vi "Climber_Execute.vi"() -> ()   [LabVIEW 2020]
uses:
  Climber_Outer_Arm_Enum.ctl
  Climber_Inner_Arm_Enum.ctl
  <vilib>/Rock Robotics/WPI/Solenoid/WPI_SolenoidValue.ctl
  <vilib>/Rock Robotics/WPI/DriverStation/WPI_DriverStationRobotMode2.ctl
  Climber_Cluster.ctl
  Climber_Control_States.ctl
  Globals/Climber_Globals.vi
  Globals/Sensor_Values.vi
  Globals/Calibration_And_Constant_Globals.vi
  Robot Global Data.vi
panel:
  out "inner arm pivot command":T1
  out "outer arm pivot command":T2
  out "elevator command":dbl=-1.0 format="%_4g"
  out "elevator Current Error":dbl=-236249.0 format="%_4g"
  in  "Outer_Arm_Elevator_Goal":dbl(slide) scale=0.0..354000.0
  in  "acceptable outer arm elevator error":dbl=3000.0
  in  "Zero_PID":T3={"Kp"=0.0, "Ki"=0.0, "Kd"=0.0, "N-Diff"=10, "N-Int"=20, "Int Error Window"=0.5, "Max Ouput"=1.0, "Min Output"=-1.0} {"Int Error Window" min=0.0; "N-Int" min=2; "N-Diff" min=2; "Kd" min=0.0; "Ki" min=0.0; "Kp" min=0.0}
  in  "Outer_Elevator_No_Load":T3={"Kp"=3e-05, "Ki"=0.0, "Kd"=0.0, "N-Diff"=10, "N-Int"=20, "Int Error Window"=0.5, "Max Ouput"=1.0, "Min Output"=-1.0} {"Int Error Window" min=0.0; "N-Int" min=2; "N-Diff" min=2; "Kd" min=0.0; "Ki" min=0.0; "Kp" min=0.0}
  in  "Disable_Outer_Arm_Elevator_Limit_Safeties":bool
  in  "Outer_Arm_Elevator_Lower_Limit":dbl
  in  "Outer_Arm_Elevator_Upper_Limit":dbl=354000.0
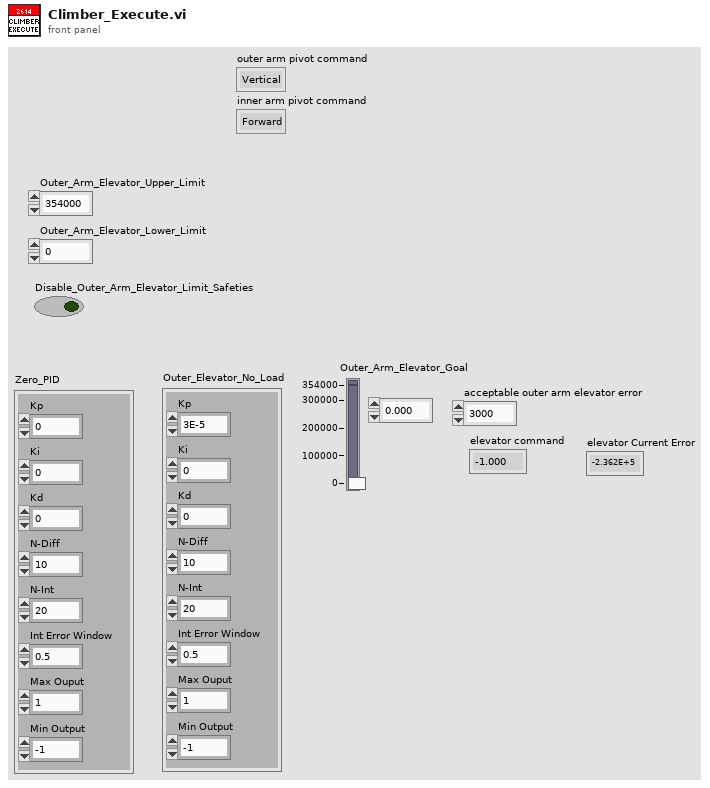
[diagram p1: front panel]
types:
  T1 = typedef "Climber_Inner_Arm_Enum.ctl" = enum16{"Forward", "Back"}
  T2 = typedef "Climber_Outer_Arm_Enum.ctl" = enum16{"Vertical", "Back"}
  T3 = cluster{"Kp":dbl, "Ki":dbl, "Kd":dbl, "N-Diff":i32, "N-Int":i32, "Int Error Window":dbl, "Max Ouput":dbl, "Min Output":dbl}
  T4 = typedef "WPI_DriverStationRobotMode2.ctl" = enum16{"Autonomous Disabled", "Autonomous Enabled", "Teleop Disabled", "Teleop Enabled", "Disconnected", "Finish", "Test Disabled", "Test Enabled", "Emergency Stopped"}
  T5 = typedef "WPI_SolenoidValue.ctl" = enum16{"No_Change", "Off", "On", "Forward", "Reverse"}
  T6 = typedef "Climber_Cluster.ctl" = cluster{"Control_State":T7, "Outer_Arm_Elevator_Throttle":dbl, "Enable_Climber_Sequence":bool, "Parameters":dbl[], "Auto_Notifier":refnum<notifier>, "Step":i32, "Advance_Sequencer_Step":bool, "Outer_Arm_Pivot_Back":bool, "Inner_Arm_Pivot_Back":bool, "Inner_Arm_Pivot_Forward":bool, "Outer_Arm_Pivot_To_Vertical":bool}
  T7 = typedef "Climber_Control_States.ctl" = enum16{"No-Op", "Manual", "Climbing_Sequence", "Tune_PID", "Command_MoveArmsToSafety"}
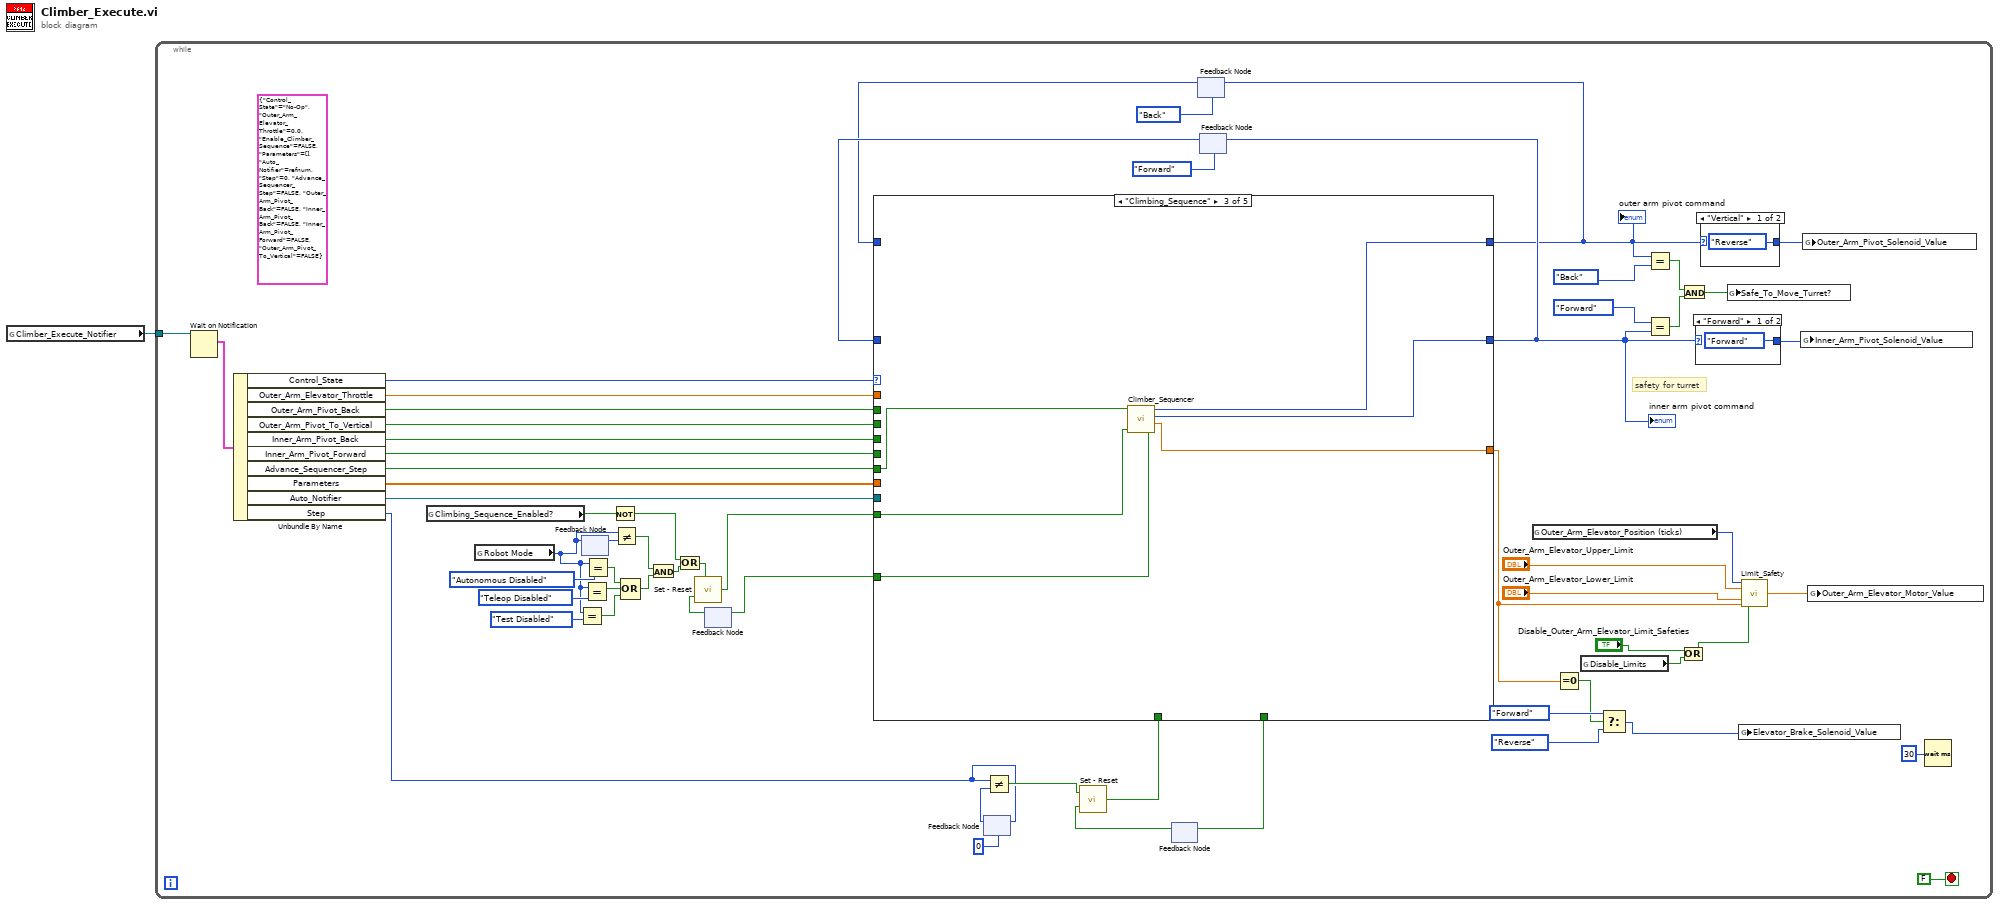
[diagram p0: block diagram]
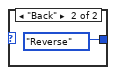
[diagram p2: hidden frame]
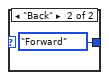
[diagram p3: hidden frame]
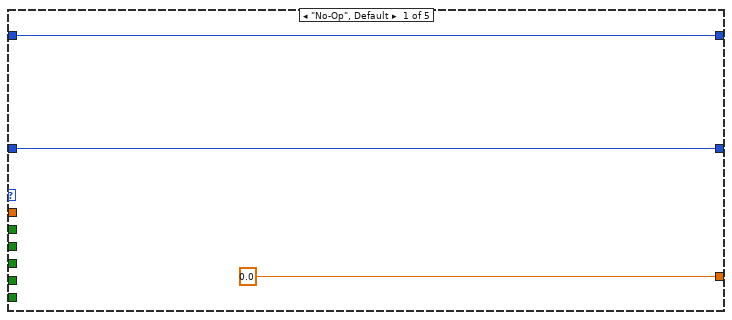
[diagram p4: hidden frame]
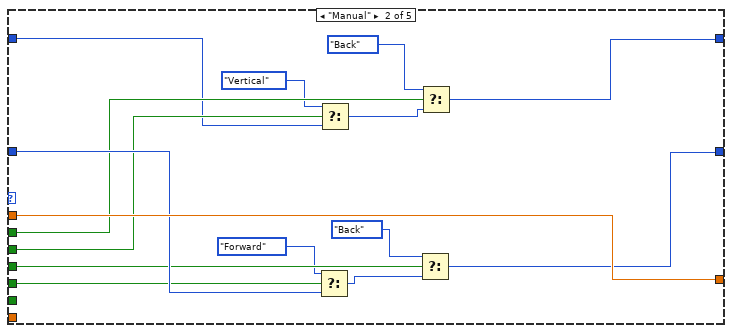
[diagram p5: hidden frame]
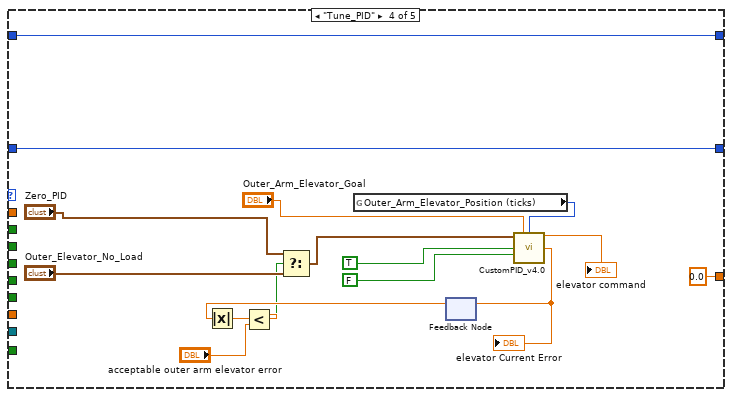
[diagram p6: hidden frame]
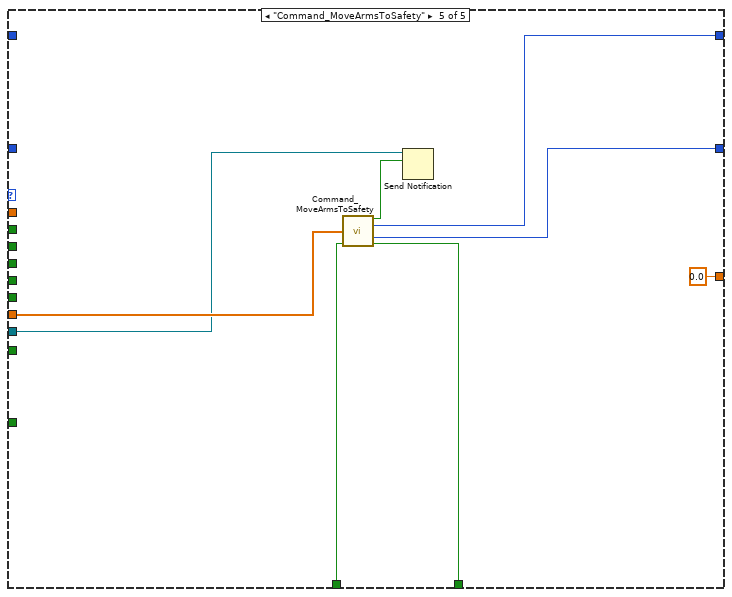
[diagram p7: hidden frame]
diagram:
  n1 = global read "Climber_Globals.vi" "Climber_Execute_Notifier"() -> (w1:refnum<notifier>)
  n2 = while {
    tunnel: w1 -> [w63]
    stop <- FALSE stop-if-true
    (unwired) T6 {"Control_State"=enum."No-Op", "Outer_Arm_Elevator_Throttle"=0.0, "Enable_Climber_Sequence"=FALSE, "Parameters"=[], "Auto_Notifier"=refnum, "Step"=0, "Advance_Sequencer_Step"=FALSE, "Outer_Arm_Pivot_Back"=FALSE, "Inner_Arm_Pivot_Back"=FALSE, "Inner_Arm_Pivot_Forward"=FALSE, "Outer_Arm_Pivot_To_Vertical"=FALSE} ("notification")
    # "safety for turret"
    n3 = Wait on Notification(notifier=w63) -> (notification=w60:T6)  [unwired: 3 in, 3 out]
    n4 = Unbundle By Name(w60) -> ("Control_State"=w38:T7, "Outer_Arm_Elevator_Throttle"=w55:dbl, "Outer_Arm_Pivot_Back"=w16:bool, "Outer_Arm_Pivot_To_Vertical"=w15:bool, "Inner_Arm_Pivot_Back"=w14:bool, "Inner_Arm_Pivot_Forward"=w13:bool, "Advance_Sequencer_Step"=w36:bool, "Parameters"=w37:dbl[], "Auto_Notifier"=w39:refnum<notifier>, "Step"=w43:i32)
    n5 = global read "Climber_Globals.vi" "Climbing_Sequence_Enabled?"() -> (w21:bool)
    n6 = global read "Robot Global Data.vi" "Robot Mode"() -> (w29:T4)
    n7 = Equal?(x=w29, y=WPI_DriverStationRobotMode2."Test Disabled" ("Robot Mode")) -> (x = y?=w30:bool)
    n8 = feedback-in #1(w29) -> ()
    n9 = feedback #1() -> (w28:T4)  [unwired: 1 in]
    n10 = Equal?(x=w29, y=WPI_DriverStationRobotMode2."Teleop Disabled" ("Robot Mode")) -> (x = y?=w31:bool)
    n11 = Equal?(x=w29, y=WPI_DriverStationRobotMode2."Autonomous Disabled" ("Robot Mode")) -> (x = y?=w32:bool)
    n12 = Not(x=w21) -> (.not. x?=w19:bool)
    n13 = Not Equal?(x=w29, y=w28) -> (x != y?=w27:bool)
    n14 = Compound Arithmetic op=OR(w32, w31, w30) -> (w26:bool)
    n15 = And(x=w27, y=w26) -> (x .and. y?=w22:bool)
    n16 = Or(x=w19, y=w22) -> (x .or. y?=w20:bool)
    n17 = feedback #2() -> (w23:bool)  [unwired: 1 in]
    n18 = call "Set - Reset.vi"("Reset"=w23, "Set"=w20) -> ("Output"=w25:bool)
    n19 = feedback #3(0 ("Step")) -> (w46:i32)
    n20 = feedback-in #3(w43) -> ()
    n21 = Not Equal?(x=w43, y=w46) -> (x != y?=w44:bool)
    n22 = feedback #4() -> (w40:bool)  [unwired: 1 in]
    n23 = call "Set - Reset.vi"("Reset"=w40, "Set"=w44) -> ("Output"=w42:bool)
    n24 = feedback #5(Climber_Outer_Arm_Enum."Back") -> (w17:T2)
    n25 = feedback #6(Climber_Inner_Arm_Enum."Forward") -> (w18:T1)
    n26 = case shown="\"Climbing_Sequence\"" w38 {
      tunnel: [0.0 ("Outer_Arm_Elevator_Motor_Value") w85 w88 0.0 ("Outer_Arm_Elevator") 0.0 ("Outer_Arm_Elevator")] -> w54
      tunnel: w55 -> [_ w85 _ _ _]
      tunnel: w37 -> [_ _ _ _ w115]
      tunnel: w42 -> [_ _ _ _ w114]
      tunnel: [_ _ _ _ w113] -> w41
      tunnel: w39 -> [_ _ _ _ w112]
      tunnel: w36 -> [_ _ w90 _ _]
      tunnel: w25 -> [_ _ w91 _ _]
      tunnel: [_ _ w89 _ _] -> w24
      tunnel: w18 -> [w68 w84 _ w92 _]
      tunnel: w17 -> [w69 w76 _ w93 _]
      tunnel: [w69 w75 w86 w93 w108] -> w5
      tunnel: [w68 w80 w87 w92 w109] -> w7
      tunnel: w16 -> [_ w78 _ _ _]
      tunnel: w15 -> [_ w79 _ _ _]
      tunnel: w14 -> [_ w81 _ _ _]
      tunnel: w13 -> [_ w83 _ _ _]
      frame "No-Op", Default {
      }
      frame "Manual" {
        n27 = Select(t=Climber_Inner_Arm_Enum."Forward", s=w83, f=w84) -> (s? t:f=w82:T1)
        n28 = Select(t=Climber_Outer_Arm_Enum."Vertical", s=w79, f=w76) -> (s? t:f=w77:T2)
        n29 = Select(t=Climber_Inner_Arm_Enum."Back", s=w81, f=w82) -> (s? t:f=w80:T1)
        n30 = Select(t=Climber_Outer_Arm_Enum."Back", s=w78, f=w77) -> (s? t:f=w75:T2)
      }
      frame "Climbing_Sequence" {
        n31 = call "Climber_Sequencer.vi"("Reset_Entire_Sequence"=w91, "Controller_Advance_Step"=w90) -> ("Sequence_Reset"=w89:bool, "Outer_Arm_Elevator"=w88:dbl, "Inner_Arm_Pneumatic"=w87:T1, "Outer_Arm_Pneumatic"=w86:T2)  [unwired: 2 in]
      }
      frame "Tune_PID" {
        n32 = global read "Sensor_Values.vi" "Outer_Arm_Elevator_Position (ticks)"() -> (w105:i32)
        n33 = feedback #7() -> (w101:dbl)  [unwired: 1 in]
        n34 = Absolute Value(x=w101) -> (abs(x)=w100:dbl)
        n35 = Less?(x=w100, y="acceptable outer arm elevator error") -> (x < y?=w97:bool)
        n36 = Select(t="Zero_PID", s=w97, f="Outer_Elevator_No_Load") -> (s? t:f=w99:T3)
        n37 = call "CustomPID_v4.0.vi"("PID Tuning Parameters"=w99, "Goal"="Outer_Arm_Elevator_Goal", "Process Variable"=w105, "Reset on Goal Change ?"=TRUE, "Use Custom Error Calculation ?"=FALSE) -> ("Command"=→"elevator command":dbl, "Current Error"=w103:dbl)  [unwired: 7 in, 2 out]
        "elevator Current Error" <- w103
        n38 = feedback-in #7(w103) -> ()
      }
      frame "Command_MoveArmsToSafety" {
        n39 = call "Command_MoveArmsToSafety.vi"("Parameters"=w115, "Startup"=w114) -> ("Completed"=w110:bool, "Outer_Arm_Pneumatic"=w108:T2, "Inner_Arm_Pneumatic"=w109:T1, "Reinit"=w113:bool)  [unwired: 10 in]
        n40 = Send Notification(notification=w110, notifier=w112) -> ()  [unwired: 1 in, 2 out]
      }
    }
    "outer arm pivot command" <- w5
    "inner arm pivot command" <- w7
    n41 = feedback-in #2(w24) -> ()
    n42 = feedback-in #4(w41) -> ()
    n43 = feedback-in #5(w5) -> ()
    n44 = feedback-in #6(w7) -> ()
    n45 = global read "Sensor_Values.vi" "Outer_Arm_Elevator_Position (ticks)"() -> (w50:i32)
    n46 = Equal To 0?(x=w54) -> (x = 0?=w57:bool)
    n47 = global read "Calibration_And_Constant_Globals.vi" "Disable_Limits"() -> (w49:bool)
    n48 = Select(t=WPI_SolenoidValue."Forward" ("Air_Brake_Solenoid_Value"), s=w57, f=WPI_SolenoidValue."Reverse" ("Air_Brake_Solenoid_Value")) -> (s? t:f=w56:T5)
    n49 = Equal?(x=w5, y=Climber_Outer_Arm_Enum."Back") -> (x = y?=w12:bool)
    n50 = Equal?(x=Climber_Inner_Arm_Enum."Forward", y=w7) -> (x = y?=w11:bool)
    n51 = Or(x="Disable_Outer_Arm_Elevator_Limit_Safeties", y=w49) -> (x .or. y?=w47:bool)
    n52 = And(x=w12, y=w11) -> (x .and. y?=w10:bool)
    n53 = case shown="\"Forward\"" w7 {
      tunnel: [WPI_SolenoidValue."Forward" ("Inner_Arm_Pivot_Solenoid_Value") WPI_SolenoidValue."Reverse" ("Inner_Arm_Pivot_Solenoid_Value")] -> w6
      frame "Forward" {
      }
      frame "Back" {
      }
    }
    n54 = case shown="\"Vertical\"" w5 {
      tunnel: [WPI_SolenoidValue."Reverse" ("Outer_Arm_Pivot_Solenoid_Value") WPI_SolenoidValue."Forward" ("Outer_Arm_Pivot_Solenoid_Value")] -> w4
      frame "Vertical" {
      }
      frame "Back" {
      }
    }
    n55 = global write "Sensor_Values.vi" "Safe_To_Move_Turret?"(w10) -> ()
    n56 = global write "Climber_Globals.vi" "Elevator_Brake_Solenoid_Value"(w56) -> ()
    n57 = call "Limit_Safety.vi"("Sensor_Value"=w50, "Upper_Limit"="Outer_Arm_Elevator_Upper_Limit", "Lower_Limit"="Outer_Arm_Elevator_Lower_Limit", "Outer_Arm_Pivot_Throttle"=w54, "Disable_Limit_Safeties"=w47) -> ("Corrected Output"=w53:dbl)  [unwired: 10 in]
    n58 = global write "Climber_Globals.vi" "Inner_Arm_Pivot_Solenoid_Value"(w6) -> ()
    n59 = global write "Climber_Globals.vi" "Outer_Arm_Pivot_Solenoid_Value"(w4) -> ()
    n60 = global write "Climber_Globals.vi" "Outer_Arm_Elevator_Motor_Value"(w53) -> ()
    n61 = Wait (ms)(milliseconds to wait=u32 30) -> ()  [unwired: 1 out]
  }
